vi "chanDesc.vi"(1 "dimensions":i64[](array[numeric])=[1399090569999999999, -1], 2 "values":T1(array[cluster]), 3 "label":string="parms") -> (0 "JSON string":string="{\"label\":\"parms\",\"values\":{\"ChanDesc\":[{\"name\":\"Alpha\",\"active\":1},{\"name\":\"Bravo\",\"active\":1},{\"name\":\"Charlie\",\"active\":1}]}}")   [LabVIEW 2014]
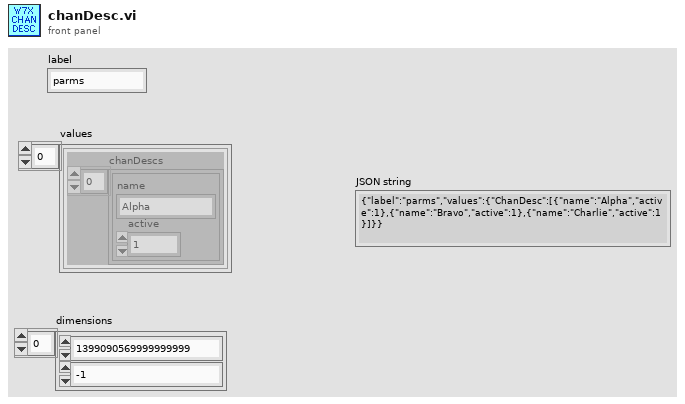
[diagram p1: front panel]
types:
  T1 = cluster{"chanDescs":cluster{"name":string, "active":i32}[]}[]
  T2 = cluster{"label":string, "values":cluster{"chanDescs":cluster{"name":string, "active":i32}[]}[], "dimensions":i64[]}
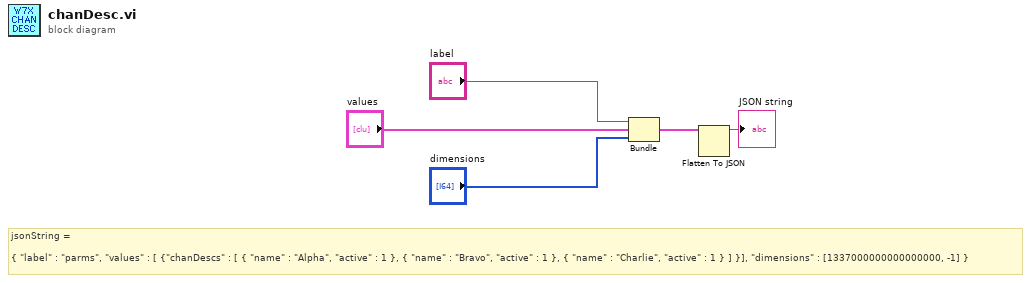
[diagram p0: block diagram]
diagram:
  # "jsonString = \n\n{ \"label\" : \"parms\", \"values\" : [ {\"chanDescs\" : [ { \"name\" : \"Alpha\", \"active\" : 1 }, { \"name\" : \"Bravo\", \"active\" : 1 }, { \"name\" : \"Charlie\", \"active\" : 1 } ] }], \"dimensions\" : [1337000000000000000, -1] }"
  n1 = Bundle("label"="label", "values"="values", "dimensions"="dimensions") -> (w4:T2)  [unwired: 1 in]
  n2 = Flatten To JSON(anything=w4) -> (JSON string=→"JSON string":string)  [unwired: 2 in, 1 out]
